vi "VisualsOfCToF.vi"() -> ()   [LabVIEW 2020]
panel:
  out "Tf":dbl(slide) scale=0.0..500.0
  in  "Tc":dbl(slide) scale=0.0..100.0
  out "Tf":dbl
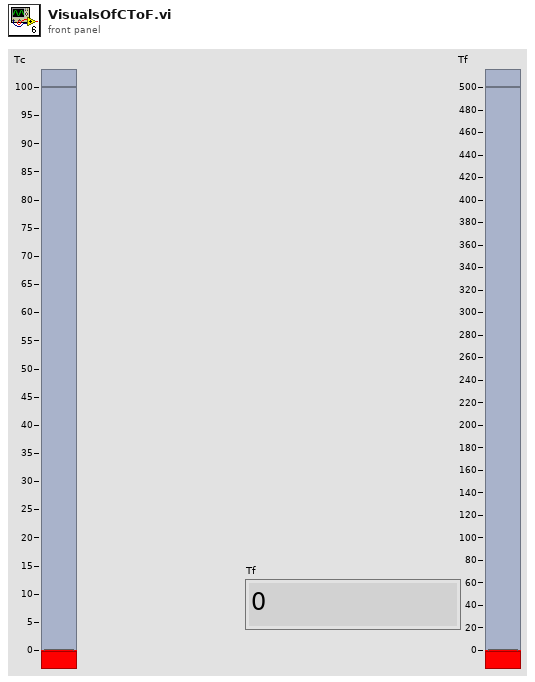
[diagram p1: front panel]
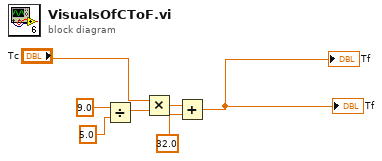
[diagram p0: block diagram]
diagram:
  n1 = Divide(x=9.0, y=5.0 ("x")) -> (x/y=w5:dbl)
  n2 = Multiply(x="Tc", y=w5) -> (x*y=w4:dbl)
  n3 = Add(x=w4, y=32.0 ("x")) -> (x+y=→"Tf" →"Tf":dbl)
